vi "Single_Cell_HPPC_Test.vi"() -> ()   [LabVIEW 2020]
panel:
  in  "Current Cutoff":dbl
  in  "Current Setpoint":dbl format="%#.6g"
  in  "Charge_B\n Voltage Setpoint":dbl format="%#.6g"
  in  "how many loops":i32
  in  "Output Safety":T1
  in  "Discharge\n time B":dbl
  in  "Discharge time A":dbl
  in  "Charge\n time A":dbl
  out "PS error out":errorcluster
  out "PS VIS resource name out":refnum<visa-resource-name>
  out "data task error out":errorcluster
  out "data task out":refnum<k21>
  in  "Wait_C time":dbl
  in  "Discharge_B Current Cutoff":dbl
  in  "Discharge_B Current Setpoint 3":dbl format="%#.6g"
  in  "Discharge_B Voltage Setpoint":dbl format="%#.6g"
  in  "Wait_B time":dbl
  in  "Charge_A Current Cutoff 2":dbl
  in  "Charge_A Current Setpoint 2":dbl format="%#.6g"
  in  "Charge_A \nVoltage Setpoint":dbl format="%#.6g"
  in  "Wait_A time":dbl
  in  "Starting Cycle":i32
  in  "Batteryname":string
  in  "data task error in":errorcluster
  in  "PS error in":errorcluster
  in  "Filepath":path=path "C:/Users/ga11/Desktop/VI/results/3PtestCharge.lvm" caption="Filename"
  in  "Discharge_A Current Cutoff":dbl
  in  "Discharge_A Current Setpoint":dbl format="%#.6g"
  in  "Discharge_A Voltage Setpoint":dbl format="%#.6g"
  in  "PS VISA in":refnum<visa-resource-name>
  in  "Data Task in":refnum<k21>
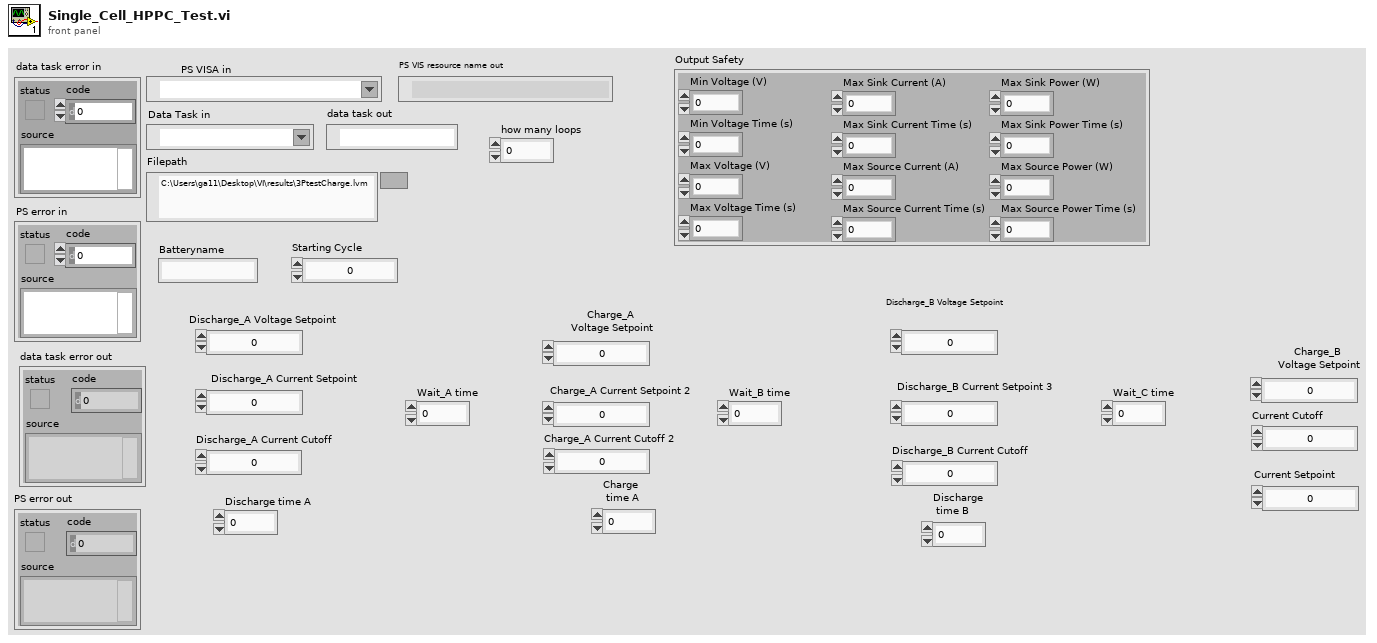
[diagram p1: front panel]
types:
  T1 = cluster{"Min Voltage (V)":dbl, "Min Voltage Time (s)":dbl, "Max Voltage (V)":dbl, "Max Voltage Time (s)":dbl, "Max Sink Current (A)":dbl, "Max Sink Current Time (s)":dbl, "Max Source Current (A)":dbl, "Max Source Current Time (s)":dbl, "Max Sink Power (W)":dbl, "Max Sink Power Time (s)":dbl, "Max Source Power (W)":dbl, "Max Source Power Time (s)":dbl}
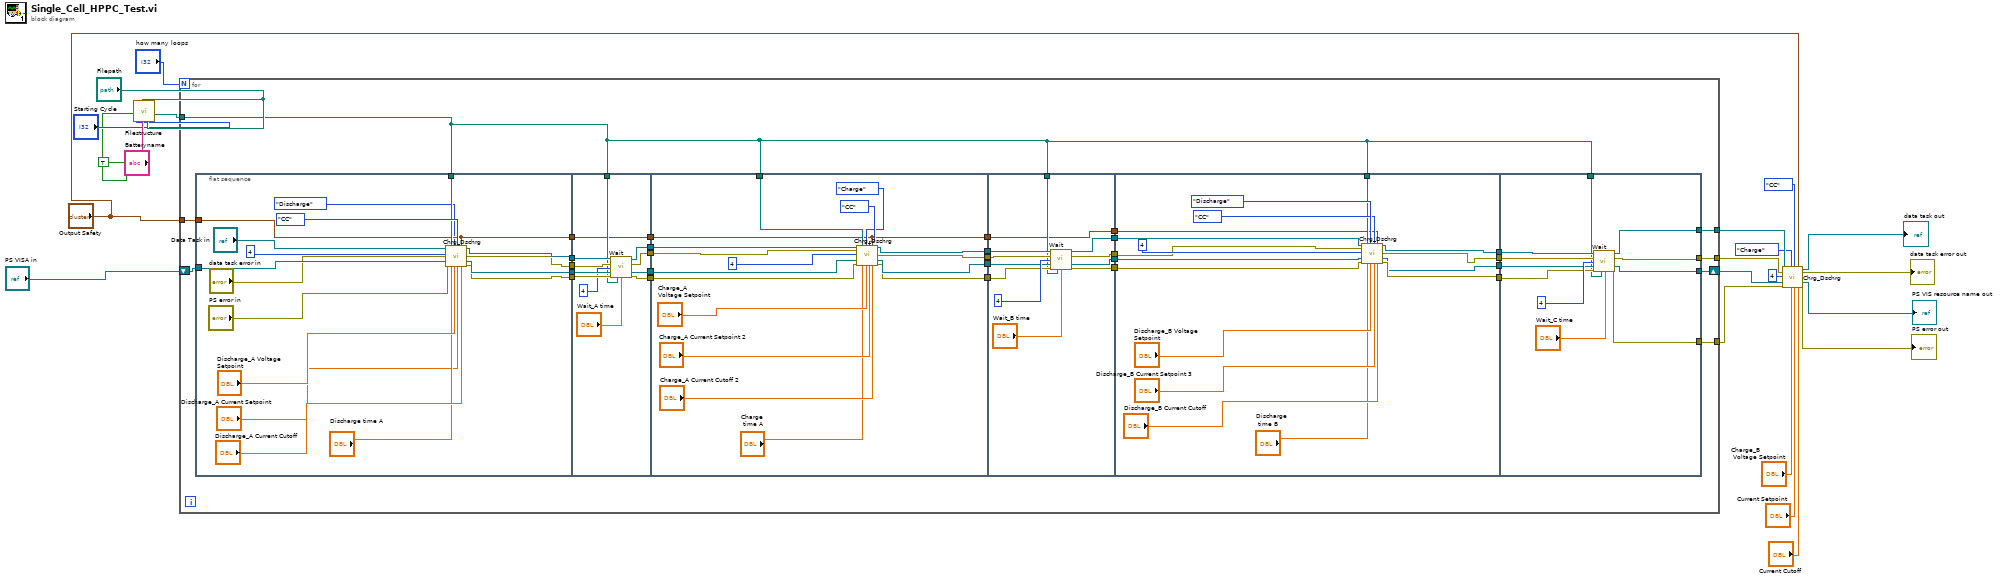
[diagram p0: block diagram]
diagram:
  n1 = call "Filestructure.vi"("Discharge filepath"="Filepath", "Batteryname"="Batteryname", "Charge filepath"="Filepath", "In for loop"=TRUE, "Starting Cycle"="Starting Cycle") -> ("DischargeCyclePath"=w17:path)  [unwired: 2 in, 4 out]
  n2 = for {
    N: "how many loops" -> [_]
    tunnel: [w32] -> w13
    tunnel: [w31] -> w14
    tunnel: [w29] -> w15
    shift-right: [w30] -> w12
    shift-left: "PS VISA in" -> [w33]
    tunnel: w17 -> [w28]
    tunnel: "Output Safety" -> [w27]
    n3 = flat-sequence {
      tunnel: w33 -> [w68]
      tunnel: [w62] -> w53
      tunnel: [w61] -> w52
      tunnel: [w60] -> w51
      tunnel: [w59] -> w50
      tunnel: w28 -> [w58]
      tunnel: w27 -> [w56]
      tunnel: [w56] -> w26
      tunnel: w53 -> [w82]
      tunnel: w52 -> [w81]
      tunnel: w51 -> [w80]
      tunnel: w50 -> [w79]
      tunnel: [w76] -> w49
      tunnel: [w75] -> w48
      tunnel: [w74] -> w47
      tunnel: [w73] -> w46
      tunnel: w28 -> [w72]
      tunnel: w26 -> [w71]
      tunnel: [w71] -> w25
      tunnel: w49 -> [w97]
      tunnel: w48 -> [w96]
      tunnel: w47 -> [w95]
      tunnel: w46 -> [w93]
      tunnel: [w89] -> w45
      tunnel: [w88] -> w44
      tunnel: [w87] -> w43
      tunnel: [w86] -> w42
      tunnel: w28 -> [w85]
      tunnel: w25 -> [w83]
      tunnel: [w83] -> w24
      tunnel: w45 -> [w109]
      tunnel: w44 -> [w108]
      tunnel: w43 -> [w107]
      tunnel: w42 -> [w106]
      tunnel: [w105] -> w41
      tunnel: [w104] -> w40
      tunnel: [w103] -> w39
      tunnel: [w102] -> w38
      tunnel: w28 -> [w101]
      tunnel: w24 -> [w100]
      tunnel: [w100] -> w23
      tunnel: w41 -> [w122]
      tunnel: w40 -> [w121]
      tunnel: w39 -> [w120]
      tunnel: w38 -> [w119]
      tunnel: [w118] -> w37
      tunnel: [w117] -> w36
      tunnel: [w116] -> w35
      tunnel: [w115] -> w34
      tunnel: w28 -> [w114]
      tunnel: w23 -> [w112]
      tunnel: w37 -> [w137]
      tunnel: w36 -> [w136]
      tunnel: w35 -> [w135]
      tunnel: w34 -> [w134]
      tunnel: [w133] -> w32
      tunnel: [w132] -> w31
      tunnel: [w131] -> w30
      tunnel: [w130] -> w29
      tunnel: w28 -> [w129]
      frame #0 {
        n4 = call "Chrg_Dschrg.vi"("Data Task in"="Data Task in", "data task error in"="data task error in", "#DAQ outputs (1-13)"=4, "PS VISA in"=w68, "PS error in"="PS error in", "DischargeCyclePath"=w58, 7:"Discharge time A", "Charge/discharge"=enum8{"Charge", "Discharge"}."Discharge", "Charge/Discharge Voltage Setpoint"="Discharge_A Voltage Setpoint", "CC or CCCV"=enum16{"CC", "CCCV"}."CC", "Current Setpoint"="Discharge_A Current Setpoint", "Output Safety"=w56, "Current Cutoff"="Discharge_A Current Cutoff") -> ("data task out"=w62:refnum<k21>, "data task error out"=w59:errorcluster, "PS VIS resource name out"=w61:refnum<visa-resource-name>, "PS error out"=w60:errorcluster)  [unwired: 3 in]
      }
      frame #1 {
        n5 = call "Wait.vi"("Data Task in"=w82, "data task error in"=w79, "#DAQ outputs (1-13)"=4, "PS VISA in"=w81, "PS error in"=w80, "Wait Filepath"=w72, "Wait time"="Wait_A time") -> ("data task out"=w76:refnum<k21>, "data task error out"=w75:errorcluster, "PS Visa Out"=w74:refnum<visa-resource-name>, "PS error out"=w73:errorcluster)  [unwired: 5 in]
      }
      frame #2 {
        n6 = call "Chrg_Dschrg.vi"("Data Task in"=w97, "data task error in"=w96, "#DAQ outputs (1-13)"=4, "PS VISA in"=w95, "PS error in"=w93, "DischargeCyclePath"=w85, 7:"Charge\n time A", "Charge/discharge"=enum8{"Charge", "Discharge"}."Charge", "Charge/Discharge Voltage Setpoint"="Charge_A \nVoltage Setpoint", "CC or CCCV"=enum16{"CC", "CCCV"}."CC", "Current Setpoint"="Charge_A Current Setpoint 2", "Output Safety"=w83, "Current Cutoff"="Charge_A Current Cutoff 2") -> ("data task out"=w89:refnum<k21>, "data task error out"=w88:errorcluster, "PS VIS resource name out"=w87:refnum<visa-resource-name>, "PS error out"=w86:errorcluster)  [unwired: 3 in]
      }
      frame #3 {
        n7 = call "Wait.vi"("Data Task in"=w109, "data task error in"=w108, "#DAQ outputs (1-13)"=4, "PS VISA in"=w107, "PS error in"=w106, "Wait Filepath"=w101, "Wait time"="Wait_B time") -> ("data task out"=w102:refnum<k21>, "data task error out"=w103:errorcluster, "PS Visa Out"=w104:refnum<visa-resource-name>, "PS error out"=w105:errorcluster)  [unwired: 5 in]
      }
      frame #4 {
        n8 = call "Chrg_Dschrg.vi"("Data Task in"=w119, "data task error in"=w120, "#DAQ outputs (1-13)"=4, "PS VISA in"=w121, "PS error in"=w122, "DischargeCyclePath"=w114, 7:"Discharge\n time B", "Charge/discharge"=enum8{"Charge", "Discharge"}."Discharge", "Charge/Discharge Voltage Setpoint"="Discharge_B Voltage Setpoint", "CC or CCCV"=enum16{"CC", "CCCV"}."CC", "Current Setpoint"="Discharge_B Current Setpoint 3", "Output Safety"=w112, "Current Cutoff"="Discharge_B Current Cutoff") -> ("data task out"=w115:refnum<k21>, "data task error out"=w116:errorcluster, "PS VIS resource name out"=w117:refnum<visa-resource-name>, "PS error out"=w118:errorcluster)  [unwired: 3 in]
      }
      frame #5 {
        n9 = call "Wait.vi"("Data Task in"=w134, "data task error in"=w135, "#DAQ outputs (1-13)"=4, "PS VISA in"=w136, "PS error in"=w137, "Wait Filepath"=w129, "Wait time"="Wait_C time") -> ("data task out"=w133:refnum<k21>, "data task error out"=w132:errorcluster, "PS Visa Out"=w131:refnum<visa-resource-name>, "PS error out"=w130:errorcluster)  [unwired: 5 in]
      }
    }
  }
  n10 = call "Chrg_Dschrg.vi"("Data Task in"=w13, "data task error in"=w14, "#DAQ outputs (1-13)"=4, "PS VISA in"=w12, "PS error in"=w15, "Charge/discharge"=enum8{"Charge", "Discharge"}."Charge", "Charge/Discharge Voltage Setpoint"="Charge_B\n Voltage Setpoint", "CC or CCCV"=enum16{"CC", "CCCV"}."CC", "Current Setpoint"="Current Setpoint", "Output Safety"="Output Safety", "Current Cutoff"="Current Cutoff") -> ("data task out"=→"data task out":refnum<k21>, "data task error out"=→"data task error out":errorcluster, "PS VIS resource name out"=→"PS VIS resource name out":refnum<visa-resource-name>, "PS error out"=→"PS error out":errorcluster)  [unwired: 5 in]
